vi "Untitled 1 (SubVI).vi"(10 "Numeric":i32, 11 "Numeric 2":dbl) -> (3 "Array":dynamicdata[](array[waveform]))   [LabVIEW 2011]
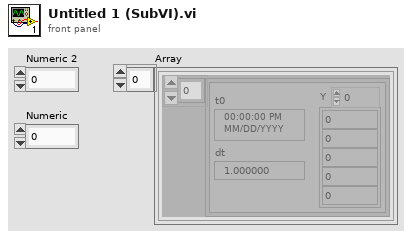
[diagram p1: front panel]
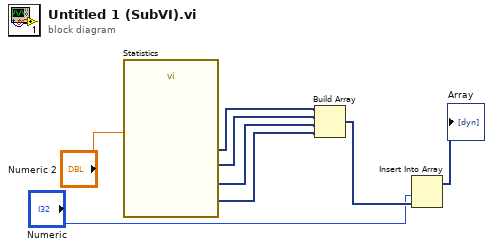
[diagram p0: block diagram]
diagram:
  n1 = call "Statistics"("Signals"="Numeric 2") -> ("Median"=w4:dynamicdata, "Variance"=w5:dynamicdata, "Minimum"=w2:dynamicdata, "Maximum"=w3:dynamicdata)  [unwired: 22 in, 1 out]
  n2 = Build Array(w5, w4, w3, w2) -> (w7:dynamicdata[])
  n3 = Insert Into Array(index="Numeric", new element=w7) -> (→"Array":dynamicdata[])  [unwired: 1 in]
